vi "UpdateTask.vi"   [LabVIEW 2012]
types:
  T1 = cluster{"Name":string, "Parameters":string[], "Start Conditional":cluster{"String":string, "avgs":cluster{"Expression":string, "Durration":dbl, "Replacement":string, "Values":dbl[]}[]}, "End Conditional":cluster{"String":string, "avgs":cluster{"Expression":string, "Durration":dbl, "Replacement":string, "Values":dbl[]}[]}, "Running":bool}
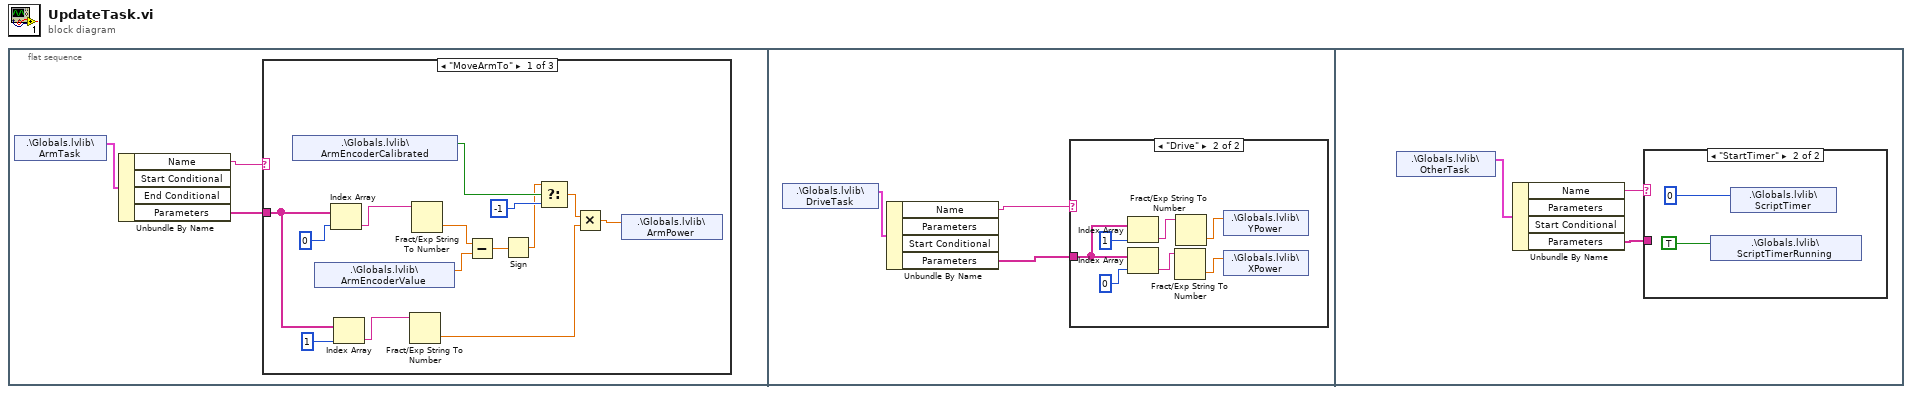
[diagram p0: block diagram]
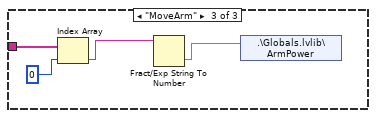
[diagram p3: hidden frame]
diagram:
  n1 = flat-sequence {
    frame #0 {
      n2 = shared-variable ".\\Globals.lvlib\\ArmTask"() -> (w3:T1)  [unwired: 1 in, 1 out]
      n3 = Unbundle By Name(w3) -> ("Name"=w2:string, "Parameters"=w1:string[])  [unwired: 2 out]
      n4 = case shown="\"MoveArmTo\"" w2 {
        tunnel: w1 -> [w13 _ w21]
        frame "MoveArmTo" {
          n5 = shared-variable ".\\Globals.lvlib\\ArmEncoderCalibrated"() -> (w15:bool)  [unwired: 1 in, 1 out]
          n6 = shared-variable ".\\Globals.lvlib\\ArmEncoderValue"() -> (w8:dbl)  [unwired: 1 in, 1 out]
          n7 = Index Array(array=w13, index=0) -> (element=w17:string)
          n8 = Index Array(array=w13, index=1) -> (element=w12:string)
          n9 = Fract/Exp String To Number(string=w12) -> (number=w9:dbl)  [unwired: 3 in, 1 out]
          n10 = Fract/Exp String To Number(string=w17) -> (number=w7:dbl)  [unwired: 3 in, 1 out]
          n11 = Subtract(x=w7, y=w8) -> (x-y=w5:dbl)
          n12 = Sign(1:w5) -> (0:w4:dbl)
          n13 = Select(t=w4, s=w15, f=-1) -> (s? t:f=w11:dbl)
          n14 = Multiply(x=w11, y=w9) -> (x*y=w10:dbl)
          n15 = shared-variable ".\\Globals.lvlib\\ArmPower"(w10) -> ()  [unwired: 1 in, 1 out]
        }
        frame Default {
        }
        frame "MoveArm" {
          n16 = Index Array(array=w21, index=0) -> (element=w19:string)
          n17 = Fract/Exp String To Number(string=w19) -> (number=w18:dbl)  [unwired: 3 in, 1 out]
          n18 = shared-variable ".\\Globals.lvlib\\ArmPower"(w18) -> ()  [unwired: 1 in, 1 out]
        }
      }
    }
    frame #1 {
      n19 = shared-variable ".\\Globals.lvlib\\DriveTask"() -> (w24:T1)  [unwired: 1 in, 1 out]
      n20 = Unbundle By Name(w24) -> ("Name"=w23:string, "Parameters"=w22:string[])  [unwired: 2 out]
      n21 = case shown="\"Drive\"" w23 {
        tunnel: w22 -> [_ w30]
        frame Default {
        }
        frame "Drive" {
          n22 = Index Array(array=w30, index=1) -> (element=w28:string)
          n23 = Index Array(array=w30, index=0) -> (element=w25:string)
          n24 = Fract/Exp String To Number(string=w25) -> (number=w27:dbl)  [unwired: 3 in, 1 out]
          n25 = Fract/Exp String To Number(string=w28) -> (number=w26:dbl)  [unwired: 3 in, 1 out]
          n26 = shared-variable ".\\Globals.lvlib\\YPower"(w26) -> ()  [unwired: 1 in, 1 out]
          n27 = shared-variable ".\\Globals.lvlib\\XPower"(w27) -> ()  [unwired: 1 in, 1 out]
        }
      }
    }
    frame #2 {
      n28 = shared-variable ".\\Globals.lvlib\\OtherTask"() -> (w34:T1)  [unwired: 1 in, 1 out]
      n29 = Unbundle By Name(w34) -> ("Name"=w33:string, "Parameters"=w32:string[])  [unwired: 2 out]
      n30 = case shown="\"StartTimer\"" w33 {
        tunnel: w32 -> [_ _]
        frame Default {
        }
        frame "StartTimer" {
          n31 = shared-variable ".\\Globals.lvlib\\ScriptTimerRunning"(TRUE) -> ()  [unwired: 1 in, 1 out]
          n32 = shared-variable ".\\Globals.lvlib\\ScriptTimer"(0) -> ()  [unwired: 1 in, 1 out]
        }
      }
    }
  }
